vi "Select COM.vi"(7 "baud rate":u32=11520, 8 "error in (no error)":errorcluster, 9 "Port Name":string, 10 "VI reference (current VI)":refnum<vi>, 11 "VISA resource name 2":refnum<visa-resource-name>) -> (0 "error out":errorcluster, 2 ".not. x?":bool, 3 "VISA resource name out":refnum<visa-resource-name>)   [LabVIEW 2017]
uses:
  <vilib>/Instr/_visa.llb/VISA Configure Serial Port (Instr).vi
panel:
  out "String":string
  in  "Blank Button":bool
  in  "VISA resource name":refnum<visa-resource-name>
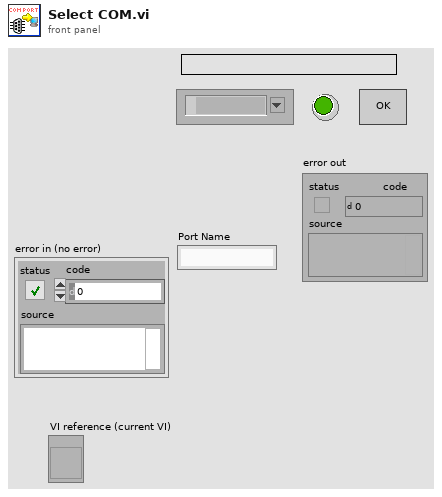
[diagram p1: front panel]
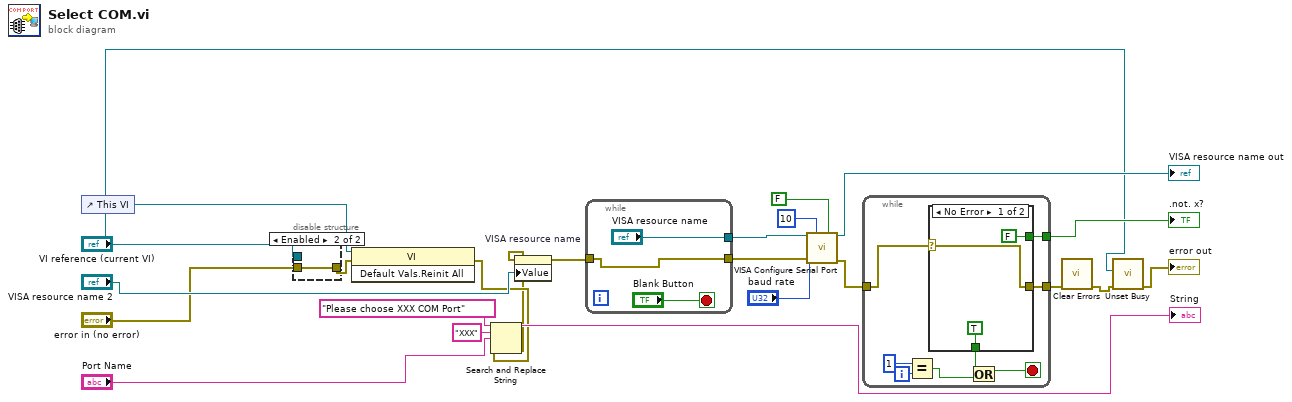
[diagram p0: block diagram]
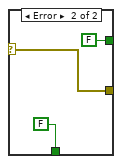
[diagram p2: hidden frame]
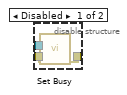
[diagram p3: hidden frame]
diagram:
  n1 = control-ref of="This VI"() -> (w23:refnum<vi>)
  n2 = disable-structure shown="Enabled" {
    disable-tunnel: "VI reference (current VI)" -> [w26 _]
    disable-tunnel: "error in (no error)" -> [w25 w27]
    disable-tunnel: [w24 w27] -> w11
    frame Disabled {
      n3 = call <vilib>:"Set Busy.vi"("error in (no error)"=w25, "VI reference (current VI)"=w26) -> ("error out"=w24:errorcluster)  [unwired: 8 in, 1 out]
    }
    frame Enabled {
    }
  }
  n4 = invoke class="VI" method="Default Vals.Reinit All"(reference=w23, error in=w11) -> (error out=w2:errorcluster)  [unwired: 1 in, 2 out]
  n5 = Search and Replace String(input string="Please choose XXX COM Port", search string="XXX", replace string="Port Name", error in=w2) -> (result string=→"String":string, error out=w1:errorcluster)  [unwired: 4 in, 2 out]
  n6 = property on="VISA resource name" class="VISAName"(error in=w1, "Value"="VISA resource name 2") -> (error out=w10:errorcluster)  [unwired: 1 in, 1 out]
  n7 = while {
    tunnel: ["VISA resource name"] -> w21
    tunnel: w10 -> [w28]
    tunnel: [w28] -> w9
    stop <- "Blank Button" stop-if-true
  }
  n8 = call-poly "VISA Configure Serial Port"("VISA resource name"=w21, "timeout (10sec)"=u32 10, "Enable Termination\nChar (T)"=FALSE ("Enable Termination\nChar (T)"), "baud rate (9600)"="baud rate", "error in (no error)"=w9) -> ("VISA resource name out"=→"VISA resource name out":refnum<visa-resource-name>, "error out"=w13:errorcluster)  [unwired: 9 in]
  n9 = while {
    tunnel: [w37] -> w14
    tunnel: w13 -> [w36]
    tunnel: [w38] -> w16
    i -> [w33]
    stop <- w34 stop-if-true
    n10 = Equal?(x=1, y=w33) -> (x = y?=w31:bool)
    n11 = case shown="No Error" w36 {
      selector: w36 -> [w41 w43]
      tunnel: [w41 w43] -> w38
      tunnel: [FALSE FALSE] -> w37
      tunnel: [TRUE FALSE] -> w35
      frame No Error {
      }
      frame Error {
      }
    }
    n12 = Or(x=w35, y=w31) -> (x .or. y?=w34:bool)
  }
  ".not. x?" <- w14
  n13 = call <vilib>:"Clear Errors.vi"("error in (no error)"=w16) -> ("error out"=w15:errorcluster)  [unwired: 5 in, 1 out]
  n14 = call <vilib>:"Unset Busy.vi"("error in (no error)"=w15, "VI reference (current VI)"="VI reference (current VI)") -> ("error out"=→"error out":errorcluster)  [unwired: 9 in]
